vi "LabVIEW Data to Python String Fast Recursion.vi"(8 "error in (no error)":errorcluster, 10 "LabVIEW Data":variant) -> (0 "error out":errorcluster, 2 "Python String":string)   [LabVIEW 2020, in "jki_python_data_tools.lvlib"]
doc: "Writes a value associated with key in a specified section of the configuration data identified by refnum. If \"key\" input is not specified, the name of the variant object is used as the key.\n\nFor example a Boolean named \"Enable\" with a value of TRUE would correspond to the key-value pair:\n\nEnable=TRUE"
uses:
  jki_python_data_tools.lvlib
panel:
  # "Copyright © 2003-2009 JKI. All rights reserved.\n\nAuthor:\nPhilippe Guerit [philippe.guerit@jameskring.com]\nJim Kring [jim.kring@jameskring.com]\n\nThis library is provided \"AS IS\" ,WITHOUT WARRANTIES OR \nCONDITIONS OF ANY KIND, either express or implied.\n\nJames Kring, Inc. -- http://www.jameskring.com"
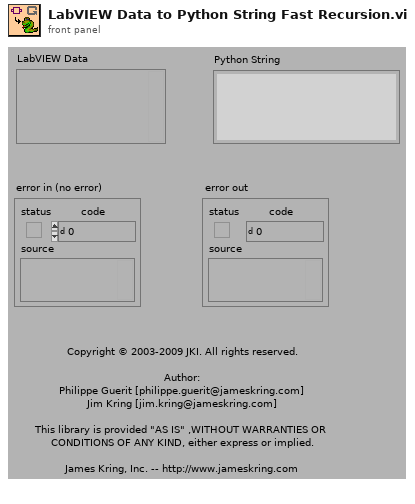
[diagram p1: front panel]
types:
  T1 = typedef "jki_python_data_tools.lvlib/Type Descriptor Enumeration__Py2LV.ctl" = enum8{"<Null>", "I8", "I16", "I32", "I64", "U8", "U16", "U32", "U64", "SGL", "DBL", "EXT", "CSG", "CDB", "CXT", "0x0F", "0x10", "0x11", "0x12", "0x13", "0x14", "Enum U8", "Enum U16", "Enum U32", "Enum U64", "SGL PQ", "DBL PQ", "EXT PQ", "CSG PQ", "CDB PQ", "CXT PQ", "0x1F", "0x20", "Boolean", "0x22", "0x23", "0x24", "0x25", "0x26", "0x27", "0x28", "0x29", "0x2A", "0x2B", "0x2C", "0x2D", "0x2E", "0x2F", "String", "0x31", "Path", "Pict", "0x34", "0x35", "0x36", "DAQ", "0x38", "0x39", "0x3A", "0x3B", "0x3C", "0x3D", "0x3E", "0x3F", "Array", "0x41", "0x42", "0x43", "0x44", "0x45", "0x46", "0x47", "0x48", "0x49", "0x4A", "0x4B", "0x4C", "0x4D", "0x4E", "0x4F", "Cluster", "0x51", "0x52", "Variant", "Waveform", "0x55", "0x56", "0x57", "0x58", "0x59", "0x5A", "0x5B", "0x5C", "0x5D", "0x5E", "0x5F", "0x60", "0x61", "0x62", "0x63", "0x64", "0x65", "0x66", "0x67", "0x68", "0x69", "0x6A", "0x6B", "0x6C", "0x6D", "0x6E", "0x6F", "Refnum"}
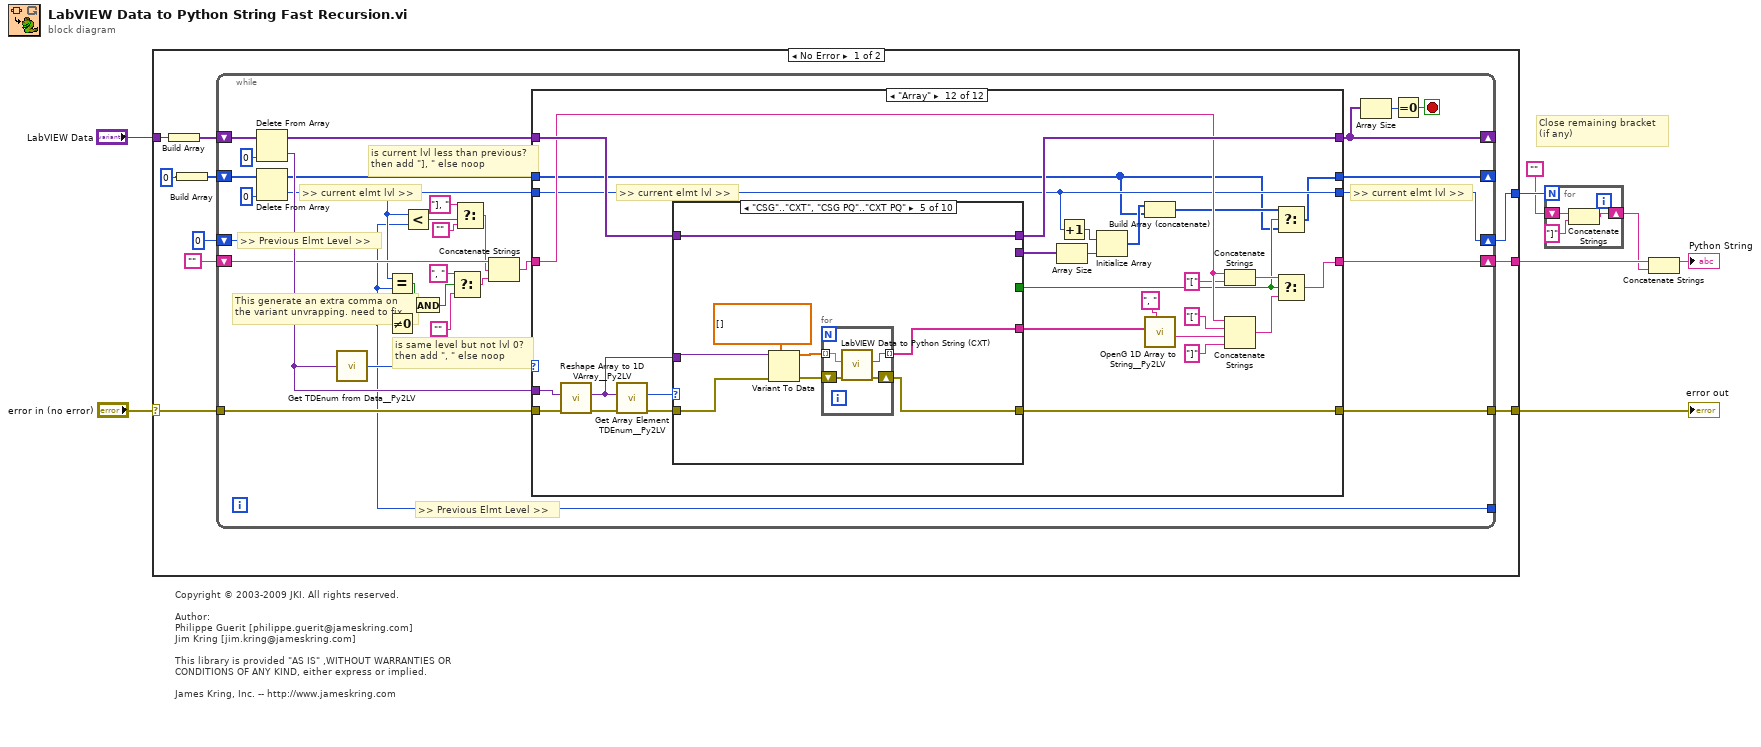
[diagram p0: block diagram]
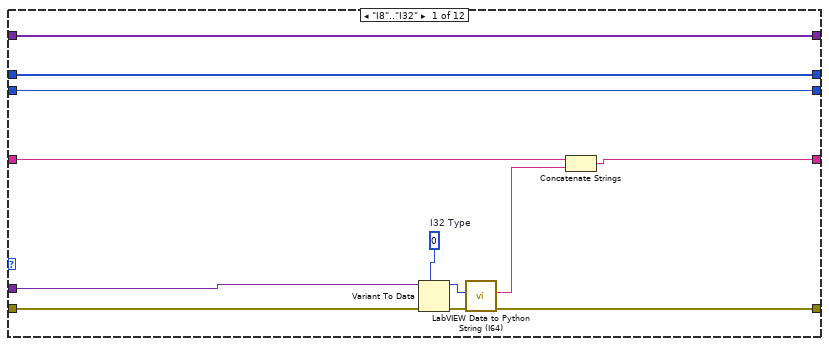
[diagram p2: hidden frame]
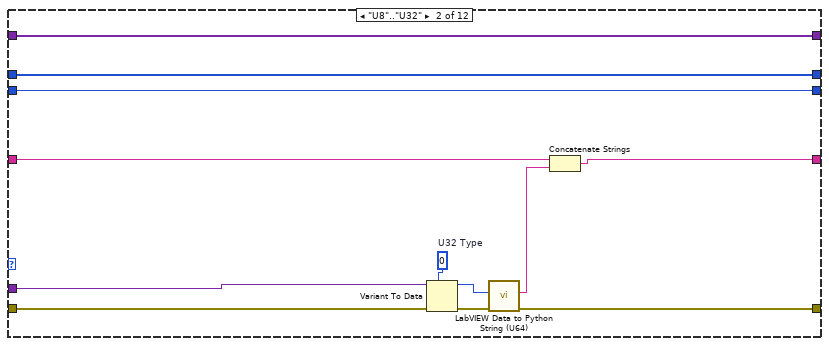
[diagram p3: hidden frame]
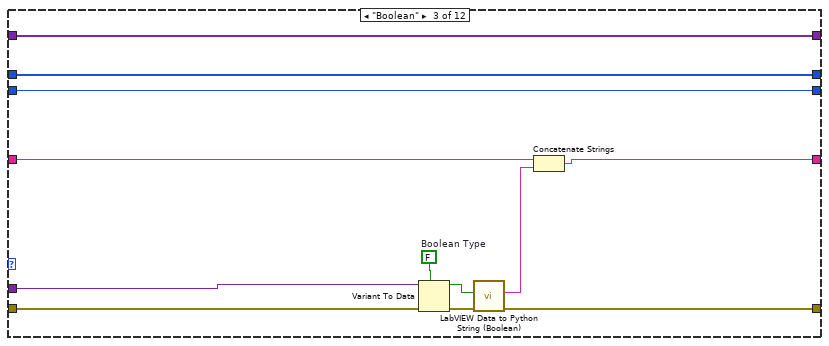
[diagram p4: hidden frame]
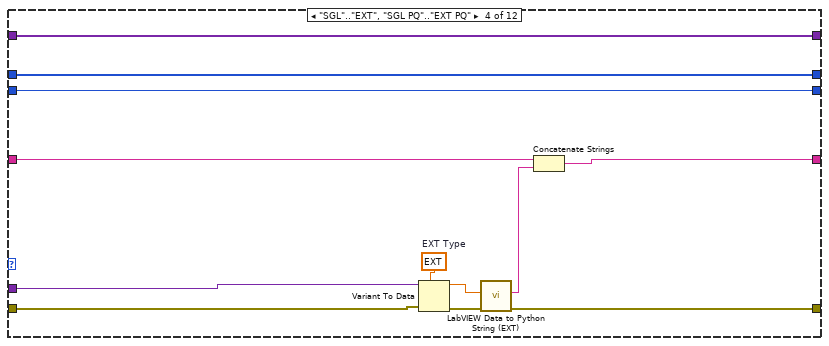
[diagram p5: hidden frame]
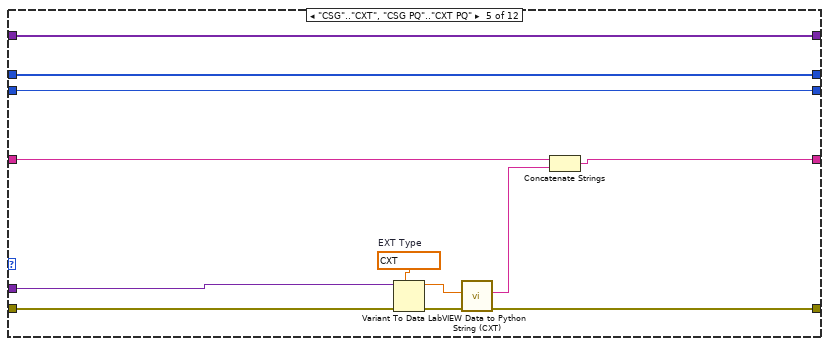
[diagram p6: hidden frame]
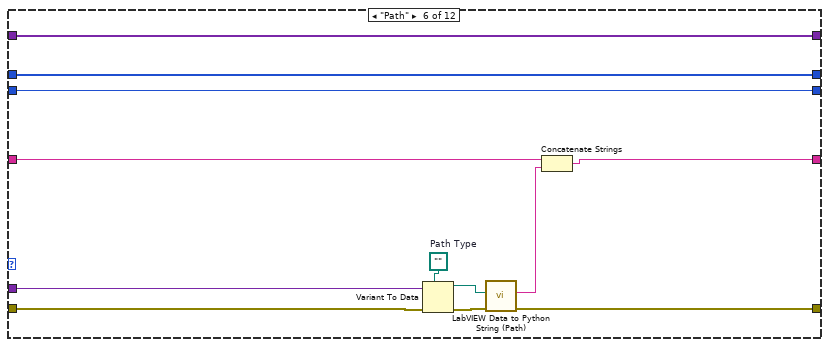
[diagram p7: hidden frame]
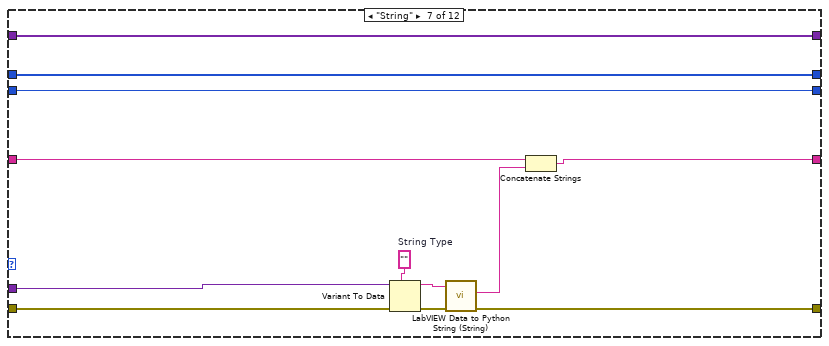
[diagram p8: hidden frame]
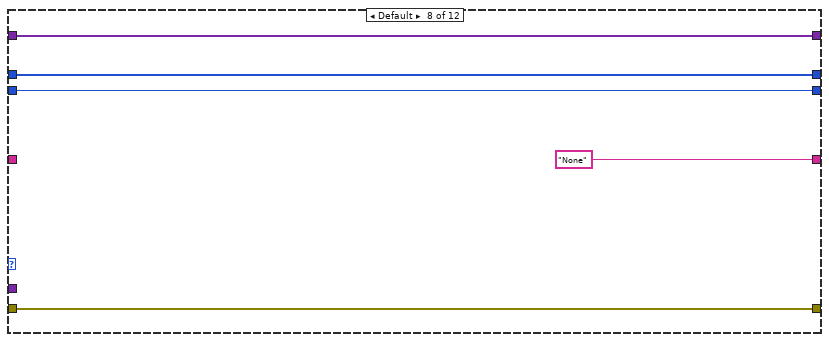
[diagram p9: hidden frame]
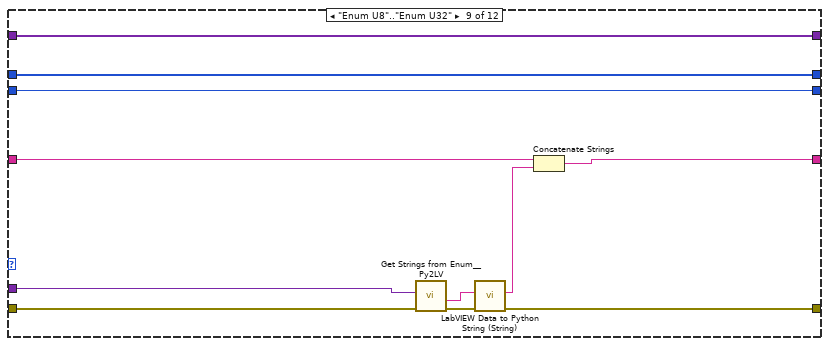
[diagram p10: hidden frame]
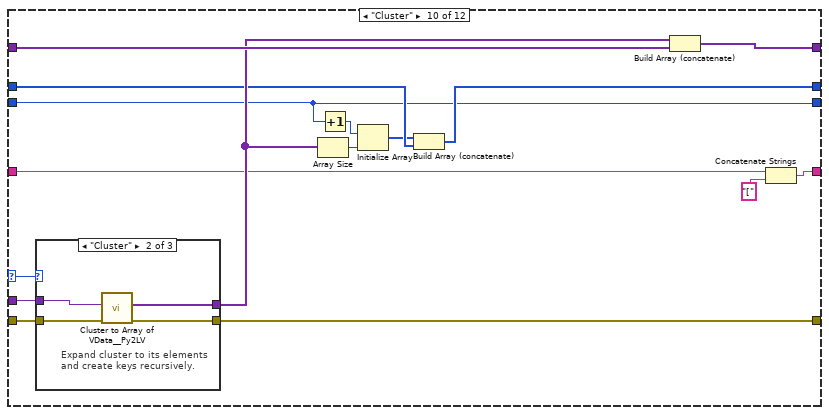
[diagram p11: hidden frame]
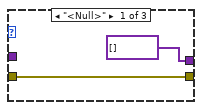
[diagram p12: hidden frame]
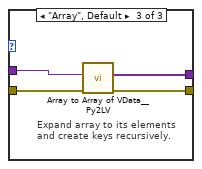
[diagram p13: hidden frame]
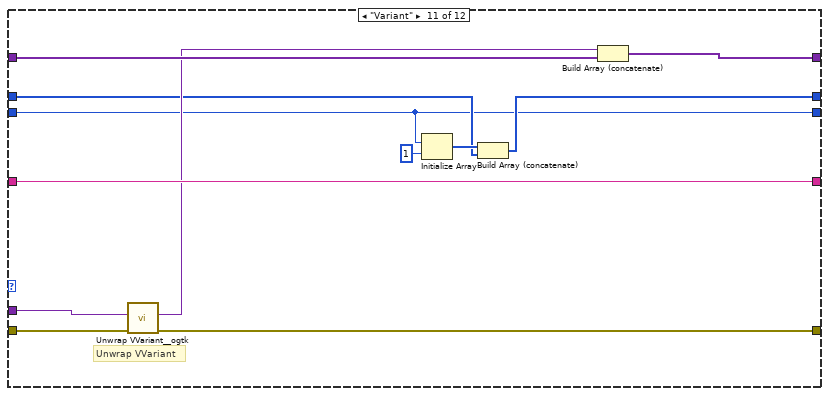
[diagram p14: hidden frame]
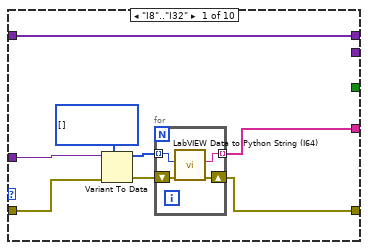
[diagram p15: hidden frame]
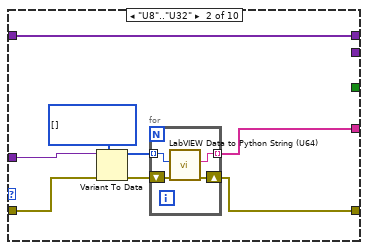
[diagram p16: hidden frame]
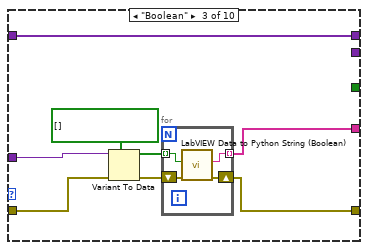
[diagram p17: hidden frame]
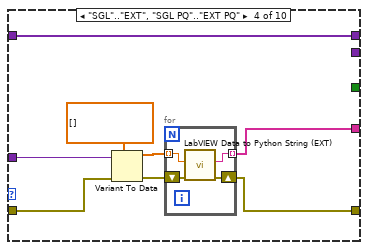
[diagram p18: hidden frame]
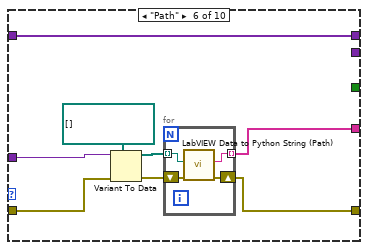
[diagram p19: hidden frame]
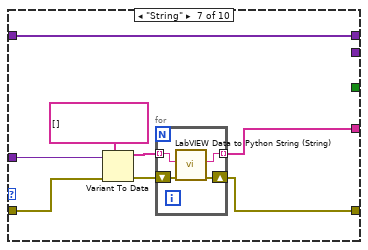
[diagram p20: hidden frame]
diagram:
  # "Copyright © 2003-2009 JKI. All rights reserved.\n\nAuthor:\nPhilippe Guerit [philippe.guerit@jameskring.com]\nJim Kring [jim.kring@jameskring.com]\n\nThis library is provided \"AS IS\" ,WITHOUT WARRANTIES OR \nCONDITIONS OF ANY KIND, either express or implied.\n\nJames Kring, Inc. -- http://www.jameskring.com"
  # "Close remaining bracket\n(if any)"
  n1 = case shown="No Error" "error in (no error)" {
    selector: "error in (no error)" -> [w18 w326]
    tunnel: [w16 w326] -> w8
    tunnel: "LabVIEW Data" -> [w15 _]
    tunnel: [w17 "None"] -> w5
    tunnel: [w9 _] -> w3
    frame No Error {
      n2 = Build Array(w15) -> (w14:variant[])
      n3 = Build Array(0) -> (w11:i32[])
      n4 = while {
        tunnel: w18 -> [w48]
        tunnel: [w47] -> w16
        shift-right: [w42] -> _
        shift-left: w14 -> [w39]
        shift-right: [w28] -> w17
        shift-left: "" -> [w32]
        shift-right: [w38] -> _
        shift-left: w11 -> [w37]
        shift-right: [w29] -> w9
        shift-left: 0 -> [w22]
        tunnel: [w22] -> _
        stop <- w40 stop-if-true
        # "This generate an extra comma on\nthe variant unvrapping. need to fix"
        # ">> current elmt lvl >>"
        # ">> Previous Elmt Level >>"
        # "is current lvl less than previous?\nthen add \"], \" else noop"
        # "is same level but not lvl 0?\nthen add \", \" else noop"
        # ">> Previous Elmt Level >>"
        # ">> current elmt lvl >>"
        n5 = Delete From Array(array=w39, index=0) -> (deleted portion=w45:variant, array with subset deleted=w43:variant[])  [unwired: 1 in]
        n6 = Delete From Array(array=w37, index=0) -> (deleted portion=w23:i32, array with subset deleted=w36:i32[])  [unwired: 1 in]
        n7 = call "Get TDEnum from Data__Py2LV.vi"("Data"=w45) -> ("Type Descriptor Enumeration"=w46:T1)  [unwired: 4 in]
        n8 = Equal?(x=w23, y=w22) -> (x = y?=w20:bool)
        n9 = Not Equal To 0?(x=w22) -> (x != 0?=w21:bool)
        n10 = Less?(x=w23, y=w22) -> (x < y?=w34:bool)
        n11 = And(x=w20, y=w21) -> (x .and. y?=w19:bool)
        n12 = Select(t=", ", s=w19, f="") -> (s? t:f=w24:string)
        n13 = Select(t="], ", s=w34, f="") -> (s? t:f=w30:string)
        n14 = Concatenate Strings(w32, w30, w24) -> (w31:string)
        n15 = case shown="\"Array\"" w46 {
          selector: w46 -> [_ _ _ _ _ _ _ _ _ w162 _ _]
          tunnel: w45 -> [w59 w71 w83 w95 w108 w119 w131 _ w147 w164 w186 w205]
          tunnel: w48 -> [w54 w70 w82 w94 w107 w118 w130 w136 w148 w163 w185 w206]
          tunnel: [w52 w63 w75 w87 w99 w111 w123 "None" w140 w150 w182 w199] -> w28
          tunnel: [w56 w67 w79 w91 w104 w115 w127 w136 w144 w159 w180 w208] -> w47
          tunnel: w43 -> [w55 w66 w78 w90 w102 w114 w126 w135 w142 w161 w184 w203]
          tunnel: [w55 w66 w78 w90 w102 w114 w126 w135 w142 w160 w183 w202] -> w42
          tunnel: w31 -> [w53 w64 w77 w89 w101 w113 w125 _ w141 w151 w182 w198]
          tunnel: w36 -> [w51 w62 w74 w86 w98 w110 w122 w134 w139 w156 w177 w188]
          tunnel: [w51 w62 w74 w86 w98 w110 w122 w134 w139 w155 w176 w187] -> w38
          tunnel: w23 -> [w49 w61 w73 w85 w97 w109 w121 w133 w138 w152 w175 w190]
          tunnel: [w49 w61 w73 w85 w97 w109 w121 w133 w138 w152 w175 w190] -> w29
          frame "I8".."I32" {
            w60 = 0  # I32 Type
            n16 = Variant To Data(error in=w54, type=w60, Variant=w59) -> (data=w58:i32, error out=w57:errorcluster)
            n17 = call "LabVIEW Data to Python String (I64).vi"("error in (no error)"=w57, "LabVIEW Data"=w58) -> ("error out"=w56:errorcluster, "Python String"=w50:string)  [unwired: 8 in]
            n18 = Concatenate Strings(w53, w50) -> (w52:string)
          }
          frame "U8".."U32" {
            w72 = u32 0  # U32 Type
            n19 = Variant To Data(error in=w70, type=w72, Variant=w71) -> (data=w68:u32, error out=w69:errorcluster)
            n20 = call "LabVIEW Data to Python String (U64).vi"("error in (no error)"=w69, "LabVIEW Data"=w68) -> ("error out"=w67:errorcluster, "Python String"=w65:string)  [unwired: 8 in]
            n21 = Concatenate Strings(w64, w65) -> (w63:string)
          }
          frame "Boolean" {
            w84 = FALSE  # Boolean Type
            n22 = Variant To Data(error in=w82, type=w84, Variant=w83) -> (data=w81:bool, error out=w80:errorcluster)
            n23 = call "LabVIEW Data to Python String (Boolean).vi"("error in (no error)"=w80, "LabVIEW Data"=w81) -> ("error out"=w79:errorcluster, "Python String"=w76:string)  [unwired: 8 in]
            n24 = Concatenate Strings(w77, w76) -> (w75:string)
          }
          frame "SGL".."EXT", "SGL PQ".."EXT PQ" {
            w96 = ext 0.0  # EXT Type
            n25 = Variant To Data(error in=w94, type=w96, Variant=w95) -> (data=w93:ext, error out=w92:errorcluster)
            n26 = call "LabVIEW Data to Python String (EXT).vi"("error in (no error)"=w92, "LabVIEW Data"=w93) -> ("error out"=w91:errorcluster, "Python String"=w88:string)  [unwired: 8 in]
            n27 = Concatenate Strings(w89, w88) -> (w87:string)
          }
          frame "CSG".."CXT", "CSG PQ".."CXT PQ" {
            w105 = cxt 0.0+0.0i  # EXT Type
            n28 = Variant To Data(error in=w107, type=w105, Variant=w108) -> (data=w103:cxt, error out=w106:errorcluster)
            n29 = call "LabVIEW Data to Python String (CXT).vi"("error in (no error)"=w106, "LabVIEW Data"=w103) -> ("error out"=w104:errorcluster, "Python String"=w100:string)  [unwired: 8 in]
            n30 = Concatenate Strings(w101, w100) -> (w99:string)
          }
          frame "Path" {
            w120 = path ""  # Path Type
            n31 = Variant To Data(error in=w118, type=w120, Variant=w119) -> (data=w117:path, error out=w116:errorcluster)
            n32 = call "LabVIEW Data to Python String (Path).vi"("error in (no error)"=w116, "LabVIEW Data"=w117) -> ("error out"=w115:errorcluster, "Python String"=w112:string)  [unwired: 8 in]
            n33 = Concatenate Strings(w113, w112) -> (w111:string)
          }
          frame "String" {
            w132 = ""  # String Type
            n34 = Variant To Data(error in=w130, type=w132, Variant=w131) -> (data=w129:string, error out=w128:errorcluster)
            n35 = call "LabVIEW Data to Python String (String).vi"("error in (no error)"=w128, "LabVIEW Data"=w129) -> ("error out"=w127:errorcluster, "Python String"=w124:string)  [unwired: 8 in]
            n36 = Concatenate Strings(w125, w124) -> (w123:string)
          }
          frame Default {
          }
          frame "Enum U8".."Enum U32" {
            n37 = call "Get Strings from Enum__Py2LV.vi"("error in (no error)"=w148, "Enum"=w147) -> ("error out"=w145:errorcluster, "String Value"=w146:string)  [unwired: 6 in, 2 out]
            n38 = call "LabVIEW Data to Python String (String).vi"("error in (no error)"=w145, "LabVIEW Data"=w146) -> ("error out"=w144:errorcluster, "Python String"=w143:string)  [unwired: 8 in]
            n39 = Concatenate Strings(w141, w143) -> (w140:string)
          }
          frame "Cluster" {
            n40 = case shown="\"Cluster\"" w162 {
              tunnel: w164 -> [_ w170 w172]
              tunnel: w163 -> [w165 w169 w171]
              tunnel: [variant[] [] w167 w174] -> w158
              tunnel: [w165 w168 w173] -> w159
              frame "<Null>" {
              }
              frame "Cluster" {
                # "Expand cluster to its elements\nand create keys recursively."
                n41 = call "Cluster to Array of VData__Py2LV.vi"("error in (no error)"=w169, "Cluster"=w170) -> ("error out"=w168:errorcluster, "Array of VData"=w167:variant[])  [unwired: 8 in]
              }
              frame "Array", Default {
                # "Expand array to its elements\nand create keys recursively."
                n42 = call "Array to Array of VData__Py2LV.vi"("error in (no error)"=w171, "MultiD Array"=w172) -> ("error out"=w173:errorcluster, "1D Array of Variants"=w174:variant[])  [unwired: 8 in]
              }
            }
            n43 = Array Size(array=w158) -> (size(s)=w157:i32)
            n44 = Increment(x=w152) -> (x+1=w154:i32)
            n45 = Initialize Array(w154, w157) -> (w153:i32[])
            n46 = Build Array (concatenate)(w153, w156) -> (w155:i32[])
            n47 = Build Array (concatenate)(w158, w161) -> (w160:variant[])
            n48 = Concatenate Strings(w151, "[" ("string")) -> (w150:string)
          }
          frame "Variant" {
            # "Unwrap VVariant"
            n49 = call <userlib>:"Unwrap VVariant__ogtk.vi"("error in (no error)"=w185, "VVariant"=w186) -> ("error out"=w180:errorcluster, "Variant"=w181:variant)  [unwired: 8 in]
            n50 = Initialize Array(w175, 1) -> (w179:i32[])
            n51 = Build Array (concatenate)(w179, w177) -> (w176:i32[])
            n52 = Build Array (concatenate)(w181, w184) -> (w183:variant[])
          }
          frame "Array" {
            # ">> current elmt lvl >>"
            n53 = call "Reshape Array to 1D VArray__Py2LV.vi"("error in (no error)"=w206, "MultiD Array"=w205) -> ("error out"=w207:errorcluster, "1D VArray"=w204:variant)  [unwired: 7 in, 1 out]
            n54 = call "Get Array Element TDEnum__Py2LV.vi"("error in (no error)"=w207, "Array"=w204) -> ("error out"=w211:errorcluster, "Element Type"=w210:T1)  [unwired: 8 in]
            n55 = case shown="\"CSG\"..\"CXT\", \"CSG PQ\"..\"CXT PQ\"" w210 {
              tunnel: w204 -> [w222 w228 w243 w254 w265 w278 w290 _ w309 w323]
              tunnel: w211 -> [w216 w229 w242 w255 w264 w279 w291 w303 w310 w324]
              tunnel: [w220 w230 w240 w253 w266 w277 w289 w300 w306 string[] []] -> w209
              tunnel: [w217 w231 w241 w252 w267 w276 w288 w303 w304 w320] -> w208
              tunnel: w203 -> [w215 w227 w239 w251 w263 w275 w287 w299 w305 w322]
              tunnel: [w215 w227 w239 w251 w263 w275 w287 w299 w305 w321] -> w202
              tunnel: [_ _ _ _ _ _ _ _ _ TRUE] -> w195
              tunnel: [_ _ _ _ _ _ _ _ _ w317] -> w191
              frame "I8".."I32" {
                n56 = Variant To Data(error in=w216, type=i32[] [], Variant=w222) -> (data=w221:i32[], error out=w218:errorcluster)
                n57 = for {
                  tunnel: w221 -> [w226] mode=indexing
                  tunnel: [w225] -> w220 mode=indexing
                  shift-right: [w223] -> w217
                  shift-left: w218 -> [w224]
                  n58 = call "LabVIEW Data to Python String (I64).vi"("error in (no error)"=w224, "LabVIEW Data"=w226) -> ("error out"=w223:errorcluster, "Python String"=w225:string)  [unwired: 8 in]
                }
              }
              frame "U8".."U32" {
                n59 = Variant To Data(error in=w229, type=u32[] [], Variant=w228) -> (data=w234:u32[], error out=w232:errorcluster)
                n60 = for {
                  tunnel: w234 -> [w238] mode=indexing
                  tunnel: [w237] -> w230 mode=indexing
                  shift-right: [w235] -> w231
                  shift-left: w232 -> [w236]
                  n61 = call "LabVIEW Data to Python String (U64).vi"("error in (no error)"=w236, "LabVIEW Data"=w238) -> ("error out"=w235:errorcluster, "Python String"=w237:string)  [unwired: 8 in]
                }
              }
              frame "Boolean" {
                n62 = Variant To Data(error in=w242, type=bool[] [], Variant=w243) -> (data=w246:bool[], error out=w244:errorcluster)
                n63 = for {
                  tunnel: w246 -> [w250] mode=indexing
                  tunnel: [w249] -> w240 mode=indexing
                  shift-right: [w247] -> w241
                  shift-left: w244 -> [w248]
                  n64 = call "LabVIEW Data to Python String (Boolean).vi"("error in (no error)"=w248, "LabVIEW Data"=w250) -> ("error out"=w247:errorcluster, "Python String"=w249:string)  [unwired: 8 in]
                }
              }
              frame "SGL".."EXT", "SGL PQ".."EXT PQ" {
                n65 = Variant To Data(error in=w255, type=ext[] [], Variant=w254) -> (data=w258:ext[], error out=w256:errorcluster)
                n66 = for {
                  tunnel: w258 -> [w262] mode=indexing
                  tunnel: [w261] -> w253 mode=indexing
                  shift-right: [w259] -> w252
                  shift-left: w256 -> [w260]
                  n67 = call "LabVIEW Data to Python String (EXT).vi"("error in (no error)"=w260, "LabVIEW Data"=w262) -> ("error out"=w259:errorcluster, "Python String"=w261:string)  [unwired: 8 in]
                }
              }
              frame "CSG".."CXT", "CSG PQ".."CXT PQ" {
                n68 = Variant To Data(error in=w264, type=cxt[] [], Variant=w265) -> (data=w270:cxt[], error out=w268:errorcluster)
                n69 = for {
                  tunnel: w270 -> [w274] mode=indexing
                  tunnel: [w273] -> w266 mode=indexing
                  shift-right: [w271] -> w267
                  shift-left: w268 -> [w272]
                  n70 = call "LabVIEW Data to Python String (CXT).vi"("error in (no error)"=w272, "LabVIEW Data"=w274) -> ("error out"=w271:errorcluster, "Python String"=w273:string)  [unwired: 8 in]
                }
              }
              frame "Path" {
                n71 = Variant To Data(error in=w279, type=path[] [], Variant=w278) -> (data=w282:path[], error out=w280:errorcluster)
                n72 = for {
                  tunnel: w282 -> [w286] mode=indexing
                  tunnel: [w285] -> w277 mode=indexing
                  shift-right: [w283] -> w276
                  shift-left: w280 -> [w284]
                  n73 = call "LabVIEW Data to Python String (Path).vi"("error in (no error)"=w284, "LabVIEW Data"=w286) -> ("error out"=w283:errorcluster, "Python String"=w285:string)  [unwired: 8 in]
                }
              }
              frame "String" {
                n74 = Variant To Data(error in=w291, type=string[] [], Variant=w290) -> (data=w294:string[], error out=w292:errorcluster)
                n75 = for {
                  tunnel: w294 -> [w298] mode=indexing
                  tunnel: [w297] -> w289 mode=indexing
                  shift-right: [w295] -> w288
                  shift-left: w292 -> [w296]
                  n76 = call "LabVIEW Data to Python String (String).vi"("error in (no error)"=w296, "LabVIEW Data"=w298) -> ("error out"=w295:errorcluster, "Python String"=w297:string)  [unwired: 8 in]
                }
              }
              frame Default {
                n77 = Initialize Array("", 0 ("dimension size")) -> (w300:string[])
              }
              frame "Enum U8".."Enum U32" {
                n78 = call "Array to Array of VData__Py2LV.vi"("error in (no error)"=w310, "MultiD Array"=w309) -> ("error out"=w308:errorcluster, "1D Array of Variants"=w307:variant[])  [unwired: 8 in]
                n79 = for {
                  tunnel: w307 -> [w313] mode=indexing
                  tunnel: [w312] -> w306 mode=indexing
                  shift-right: [w311] -> w304
                  shift-left: w308 -> [w314]
                  n80 = call "Get Strings from Enum__Py2LV.vi"("error in (no error)"=w314, "Enum"=w313) -> ("error out"=w316:errorcluster, "String Value"=w315:string)  [unwired: 6 in, 2 out]
                  n81 = call "LabVIEW Data to Python String (String).vi"("error in (no error)"=w316, "LabVIEW Data"=w315) -> ("error out"=w311:errorcluster, "Python String"=w312:string)  [unwired: 8 in]
                }
              }
              frame "Cluster" {
                n82 = call "Array to Array of VData__Py2LV.vi"("error in (no error)"=w324, "MultiD Array"=w323) -> ("error out"=w320:errorcluster, "1D Array of Variants"=w317:variant[])  [unwired: 8 in]
                n83 = Build Array (concatenate)(w317, w322) -> (w321:variant[])
              }
            }
            n84 = Array Size(array=w191) -> (size(s)=w194:i32)
            n85 = Increment(x=w190) -> (x+1=w193:i32)
            n86 = Initialize Array(w193, w194) -> (w192:i32[])
            n87 = Build Array (concatenate)(w192, w188) -> (w189:i32[])
            n88 = call "OpenG 1D Array to String__Py2LV.vi"("delimiter (Tab)"=", ", "Array of Strings"=w209) -> ("delimited string"=w213:string)  [unwired: 9 in]
            n89 = Concatenate Strings(w198, "[" ("string")) -> (w197:string)
            n90 = Concatenate Strings(w198, "[" ("string"), w213, "]" ("string")) -> (w200:string)
            n91 = Select(t=w189, s=w195, f=w188) -> (s? t:f=w187:i32[])
            n92 = Select(t=w197, s=w195, f=w200) -> (s? t:f=w199:string)
          }
        }
        n93 = Array Size(array=w42) -> (size(s)=w41:i32)
        n94 = Equal To 0?(x=w41) -> (x = 0?=w40:bool)
      }
    }
    frame Error {
    }
  }
  "error out" <- w8
  n95 = for {
    N: w3 -> [_]
    shift-right: [w329] -> w1
    shift-left: "" -> [w328]
    n96 = Concatenate Strings(w328, "]" ("t")) -> (w329:string)
  }
  n97 = Concatenate Strings(w5, w1) -> (→"Python String":string)
